vi "Embedded UI example.vi"() -> ()   [LabVIEW 2017]
panel:
  out "Total":i32
  in  "Add":bool
  in  "stop":bool
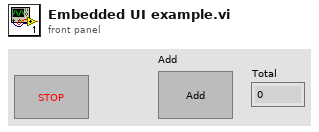
[diagram p1: front panel]
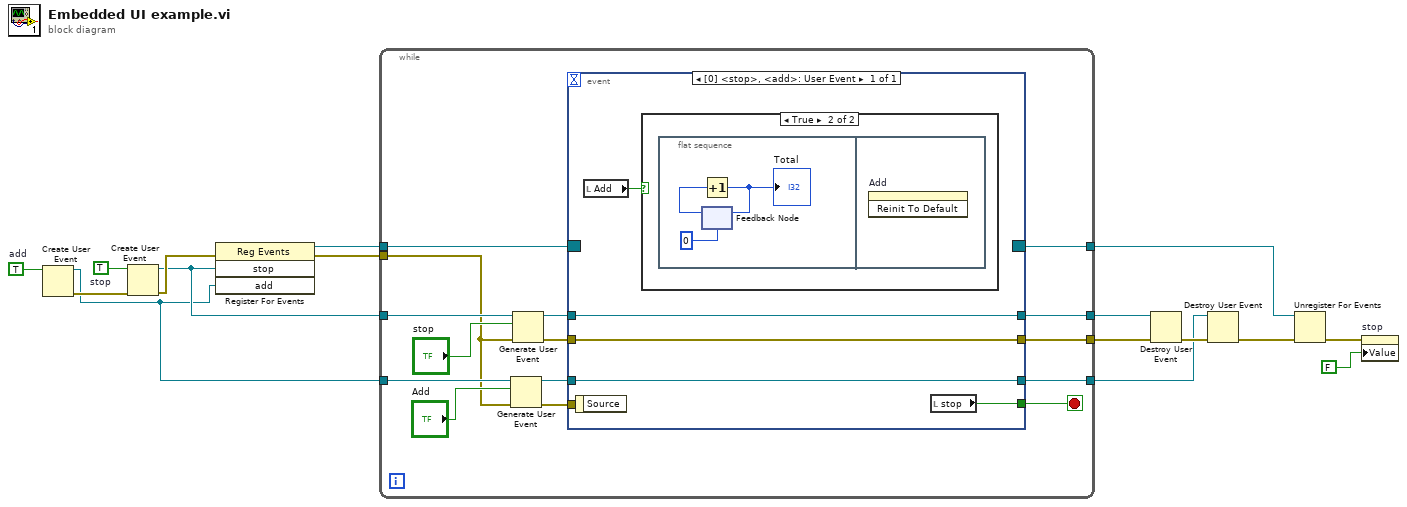
[diagram p0: block diagram]
diagram:
  w6 = TRUE  # add
  w16 = TRUE  # stop
  n1 = Create User Event(user event datatype=w6) -> (user event=w4:refnum<user-event>, error out=w5:errorcluster)  [unwired: 1 in]
  n2 = Create User Event(user event datatype=w16, error in=w5) -> (user event=w11:refnum<user-event>, error out=w13:errorcluster)
  n3 = register-events(error in=w13, w11, w4) -> (reference out=w15:refnum<event-registration>, error out=w10:errorcluster)  [unwired: 1 in]
  n4 = while {
    tunnel: w15 -> [w31]
    tunnel: [w30] -> w14
    tunnel: [w28] -> w12
    tunnel: w11 -> [w26]
    tunnel: w10 -> [w20]
    tunnel: [w23] -> w9
    tunnel: w4 -> [w22]
    tunnel: [w17] -> w1
    stop <- w29 stop-if-true
    n5 = Generate User Event(user event=w22, event data cluster="Add", error in=w20) -> (user event out=w18:refnum<user-event>, error out=w19:errorcluster)  [unwired: 1 in]
    n6 = Generate User Event(user event=w26, event data cluster="stop", error in=w20) -> (user event out=w25:refnum<user-event>, error out=w24:errorcluster)  [unwired: 1 in]
    n7 = event shown="[0] <stop>, <add>: User Event" {
      selector: w31 -> [_]
      dyn-events: [_] -> w30
      timeout: _ -> [_]
      tunnel: [w33] -> w29
      tunnel: [w36] -> w28
      tunnel: w25 -> [w36]
      tunnel: w24 -> [w35]
      tunnel: [w35] -> w23
      tunnel: w19 -> [_]
      tunnel: [w34] -> w17
      tunnel: w18 -> [w34]
      event User Event {
        n8 = event-data() -> ()  [unwired: 1 in, 1 out]
        n9 = local read "Add"() -> (w32:bool)
        n10 = case shown="True" w32 {
          frame False {
          }
          frame True {
            n11 = flat-sequence {
              frame #0 {
                n12 = feedback #1(0) -> (w38:i32)
                n13 = Increment(x=w38) -> (x+1=w39:i32)
                "Total" <- w39
                n14 = feedback-in #1(w39) -> ()
              }
              frame #1 {
                n15 = invoke on="Add" class="Bool (strict)" method="Reinit To Default"() -> ()  [unwired: 3 in, 3 out]
              }
            }
          }
        }
        n16 = local read "stop"() -> (w33:bool)
      }
    }
  }
  n17 = Destroy User Event(user event=w12, error in=w9) -> (error out=w3:errorcluster)
  n18 = Destroy User Event(user event=w1, error in=w3) -> (error out=w2:errorcluster)
  n19 = Unregister For Events(event registration refnum=w14, error in=w2) -> (error out=w7:errorcluster)
  n20 = property on="stop" class="Bool (strict)"(error in=w7, "Value"=FALSE ("stop")) -> ()  [unwired: 1 in, 2 out]
